vi "ErrorLog_SelectInitialFile.vi"(8 "error in (no error)":errorcluster, 11 "reference in":refnum<class "ErrorLog.lvclass">) -> (0 "error out":errorcluster, 3 "reference out":refnum<class "ErrorLog.lvclass">)   [LabVIEW 2014, in "ErrorLog.lvclass"]
uses:
  ErrorLog.lvclass
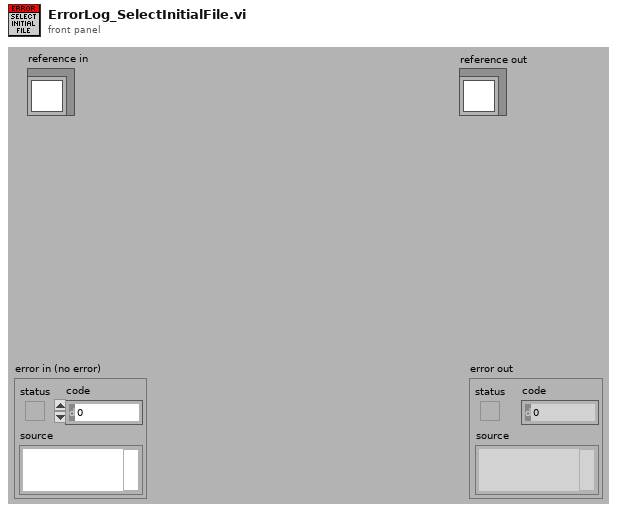
[diagram p1: front panel]
types:
  T1 = typedef "ErrorLog.lvclass/ObjectAttributes.ctl" = cluster{"ErrorFile":path, "Supress Consecutive Duplicates":bool, "Errors":string, "Quit":bool, "Errors since last call":string, "Last Recorded Error":string, "ErrorPath":path, "PossiblePaths":path[], "BaseFileName":string, "Max Log Files":i32, "ErrorFile Index":i32, "Max File Size":i64}
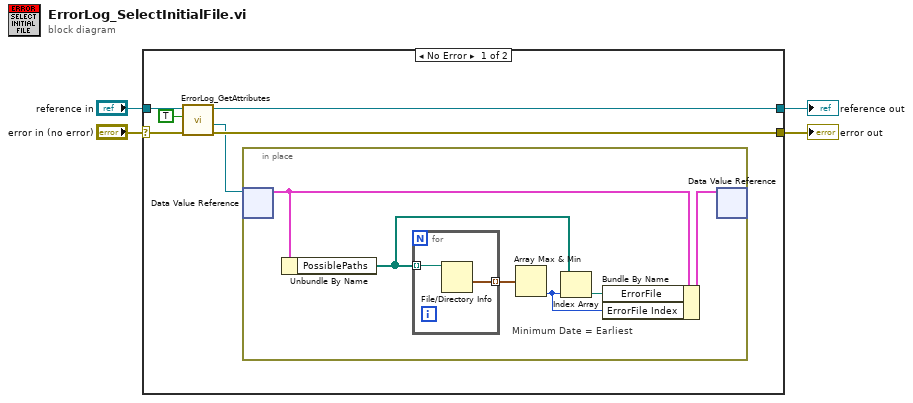
[diagram p0: block diagram]
diagram:
  n1 = case shown="No Error" "error in (no error)" {
    selector: "error in (no error)" -> [w10 w20]
    tunnel: [w9 w20] -> w3
    tunnel: [w7 w19] -> w1
    tunnel: "reference in" -> [w8 w19]
    frame No Error {
      n2 = call "ErrorLog_GetAttributes.vi"("error in (no error)"=w10, "OnlyGetDvrReference(False)"=TRUE, "reference in"=w8) -> ("error out"=w9:errorcluster, "DataRef"=w5:refnum<data-value>, "reference out"=w7:refnum<class "ErrorLog.lvclass">)  [unwired: 5 in, 1 out]
      n3 = in-place {
        # "Minimum Date = Earliest"
        n4 = in-place-dvr #1(w5) -> (w16:T1)  [unwired: 1 out]
        n5 = Unbundle By Name(w16) -> ("PossiblePaths"=w13:path[])
        n6 = for {
          tunnel: w13 -> [w18] mode=indexing
          tunnel: [w17] -> w14 mode=indexing
          n7 = File/Directory Info(path=w18) -> (last mod=w17:timestamp)  [unwired: 1 in, 6 out]
        }
        n8 = Array Max & Min(array=w14) -> (min index (indices)=w11:i32)  [unwired: 3 out]
        n9 = Index Array(array=w13, index=w11) -> (element=w12:path)
        n10 = Bundle By Name(cluster=w16, "ErrorFile"=w12, "ErrorFile Index"=w11) -> (w15:T1)
        n11 = in-place-dvr #1(w15) -> ()  [unwired: 2 out]
      }
    }
    frame Error {
    }
  }
  "error out" <- w3
  "reference out" <- w1
